vi "WriteLeftActive.vi"(8 "error in (no error)":errorcluster, 10 "Left Active":i32, 11 "EmbeddedMainUI in":refnum<class "EmbeddedMainUI.lvclass">) -> (0 "error out":errorcluster, 3 "EmbeddedMainUI out":refnum<class "EmbeddedMainUI.lvclass">)   [LabVIEW 2016, in "EmbeddedMainUI.lvclass"]
uses:
  EmbeddedMainUI.lvclass
  EmbeddedMainUI.lvclass/EmbeddedMainUI.ctl
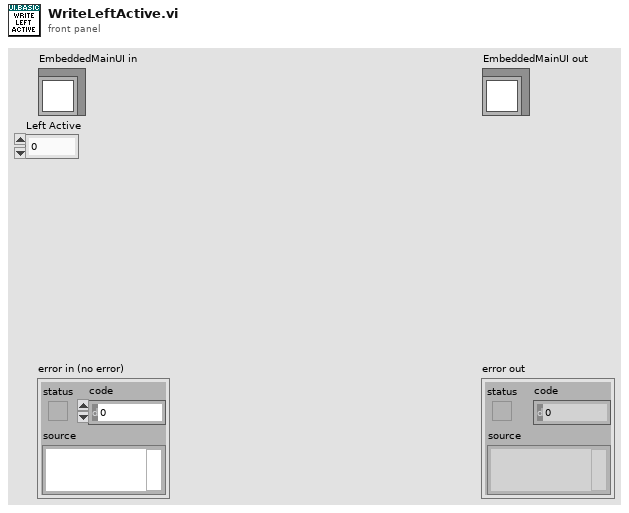
[diagram p1: front panel]
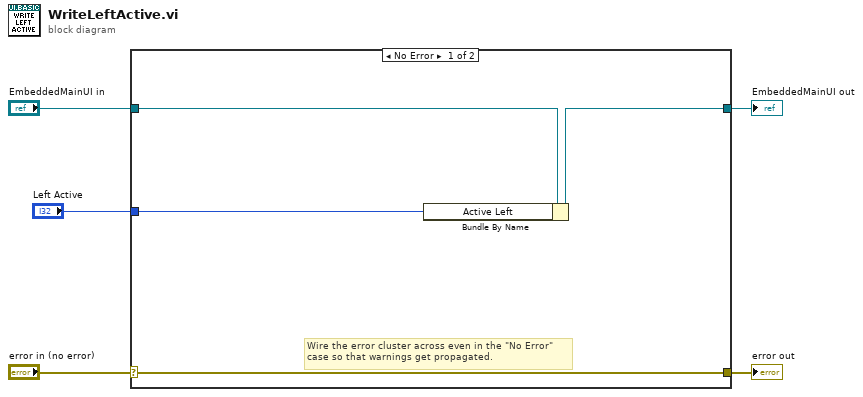
[diagram p0: block diagram]
diagram:
  n1 = case shown="No Error" "error in (no error)" {
    selector: "error in (no error)" -> [w9 w11]
    tunnel: [w9 w11] -> w4
    tunnel: [w7 w10] -> w2
    tunnel: "EmbeddedMainUI in" -> [w8 w10]
    tunnel: "Left Active" -> [w6 _]
    frame No Error {
      # "Wire the error cluster across even in the \"No Error\"\ncase so that warnings get propagated."
      n2 = Bundle By Name(cluster=w8, "Active Left"=w6) -> (w7:refnum<class "EmbeddedMainUI.lvclass">)
    }
    frame Error {
    }
  }
  "error out" <- w4
  "EmbeddedMainUI out" <- w2
